vi "Set Plot title.vi"(8 "error in":errorcluster, 10 "Title Text":string, 11 "XY Plot Title Reference":refnum<vi>) -> (0 "error out":errorcluster, 3 "XY Plot Title Reference":refnum<vi>)   [LabVIEW 2017, in "DTacq Plot Display Library.lvlib"]
uses:
  DTacq Plot Display Library.lvlib
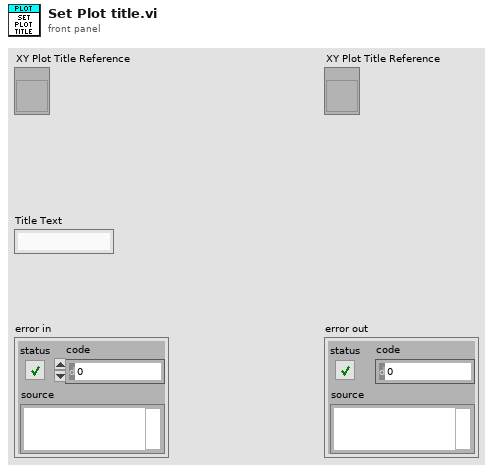
[diagram p1: front panel]
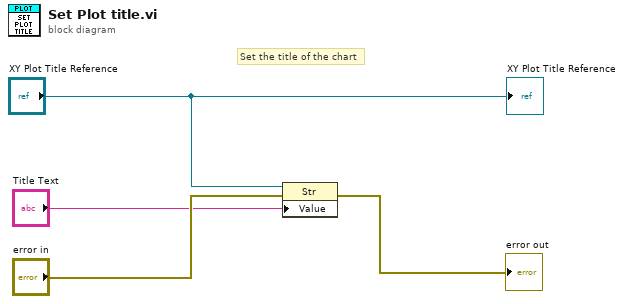
[diagram p0: block diagram]
diagram:
  # "Set the title of the chart"
  n1 = property class="Str"(reference="XY Plot Title Reference", error in="error in", "Value"="Title Text") -> (error out=→"error out":errorcluster)  [unwired: 1 out]
  "XY Plot Title Reference" <- "XY Plot Title Reference"
